vi "Build Tree From Data (Recursive).vi"(8 "error in (no error)":errorcluster, 9 "Hierarchical Data {VAT}":variant, 10 "Parent Tag (empty)":string, 11 "TreeControl Ref":refnum<vi>) -> (0 "error out":errorcluster, 1 "Leaf-Level?":bool, 3 "TreeControl Ref":refnum<vi>)   [LabVIEW 2015, in "TreeExtensions.lvlib"]
uses:
  TreeExtensions.lvlib
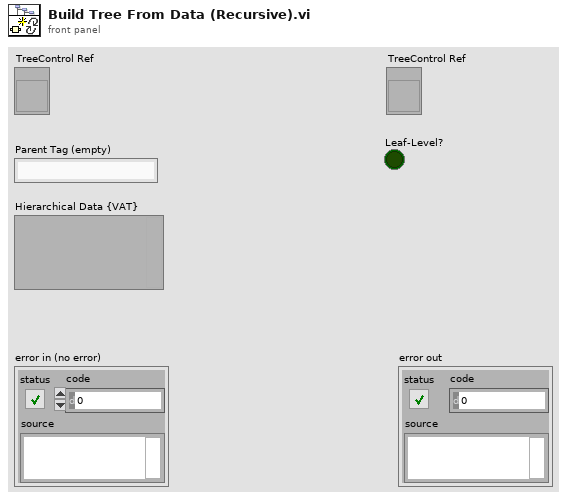
[diagram p1: front panel]
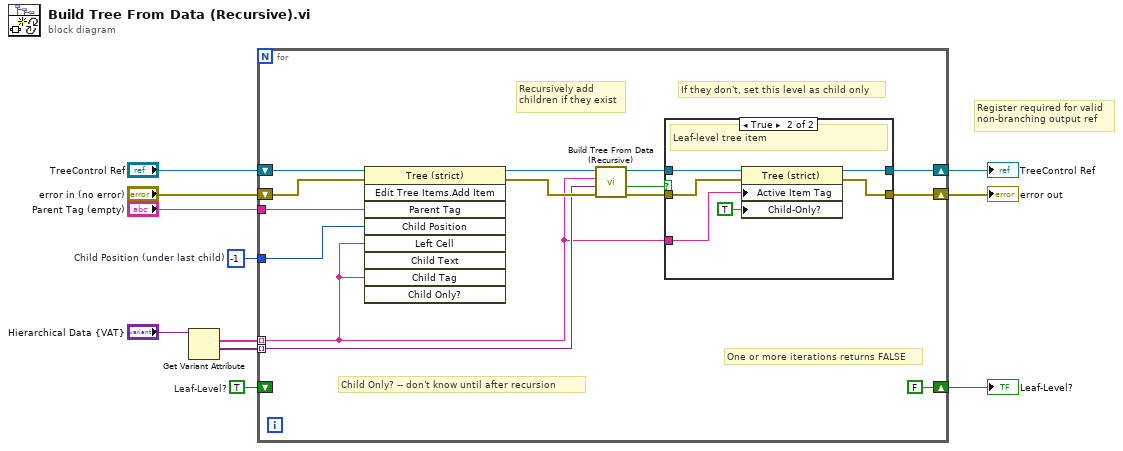
[diagram p0: block diagram]
diagram:
  w2 = TRUE  # Leaf-Level?
  w3 = -1  # Child Position (under last child)
  # "Register required for valid\nnon-branching output ref"
  n1 = Get Variant Attribute(Variant="Hierarchical Data {VAT}") -> (names=w11:string[], values=w5:variant[])  [unwired: 3 in, 2 out]
  n2 = for {
    tunnel: w5 -> [w20] mode=indexing
    shift-right: [w14] -> w9
    shift-left: "error in (no error)" -> [w24]
    tunnel: "Parent Tag (empty)" -> [w23]
    tunnel: w11 -> [w12] mode=indexing
    shift-right: [w13] -> w4
    shift-left: "TreeControl Ref" -> [w25]
    tunnel: w3 -> [w21]
    shift-right: [FALSE ("Leaf-Level?")] -> w1
    shift-left: w2 -> [_]
    # "Child Only? -- don't know until after recursion"
    # "If they don't, set this level as child only"
    # "One or more iterations returns FALSE"
    # "Recursively add\nchildren if they exist"
    n3 = invoke class="Tree (strict)" method="Edit Tree Items.Add Item"(reference=w25, error in=w24, "Parent Tag"=w23, "Child Position"=w21, "Left Cell"=w12, "Child Tag"=w12) -> (reference out=w19:refnum<vi>, error out=w22:errorcluster)  [unwired: 3 in, 7 out]
    n4 = call "Build Tree From Data (Recursive).vi"("error in (no error)"=w22, "Hierarchical Data {VAT}"=w20, "Parent Tag (empty)"=w12, "TreeControl Ref"=w19) -> ("error out"=w15:errorcluster, "Leaf-Level?"=w17:bool, "TreeControl Ref"=w16:refnum<vi>)  [unwired: 5 in]
    n5 = case shown="True" w17 {
      tunnel: w16 -> [w27 w33]
      tunnel: w15 -> [w26 w32]
      tunnel: [w26 w31] -> w14
      tunnel: [w27 w30] -> w13
      tunnel: w12 -> [_ w28]
      frame False {
        # "Not leaf-level (skip prop node call)"
      }
      frame True {
        # "Leaf-level tree item"
        n6 = property class="Tree (strict)"(reference=w33, error in=w32, "Active Item Tag"=w28, "Child-Only?"=TRUE ("Active Item:Child-Only?")) -> (reference out=w30:refnum<vi>, error out=w31:errorcluster)
      }
    }
  }
  "error out" <- w9
  "TreeControl Ref" <- w4
  "Leaf-Level?" <- w1
